vi "LV SciSDK ADD BOARD.vi"(5 "JsonFile":path, 7 "Board Model":string(combo), 8 "error in (no error)":errorcluster, 9 "handle":u64, 10 "DevicePath":string, 11 "Name":string) -> (0 "error out":errorcluster, 3 "handle":T1)   [LabVIEW 2021]
uses:
  SciSDK_Labview.lvlib
panel:
  out "Add device result":i32
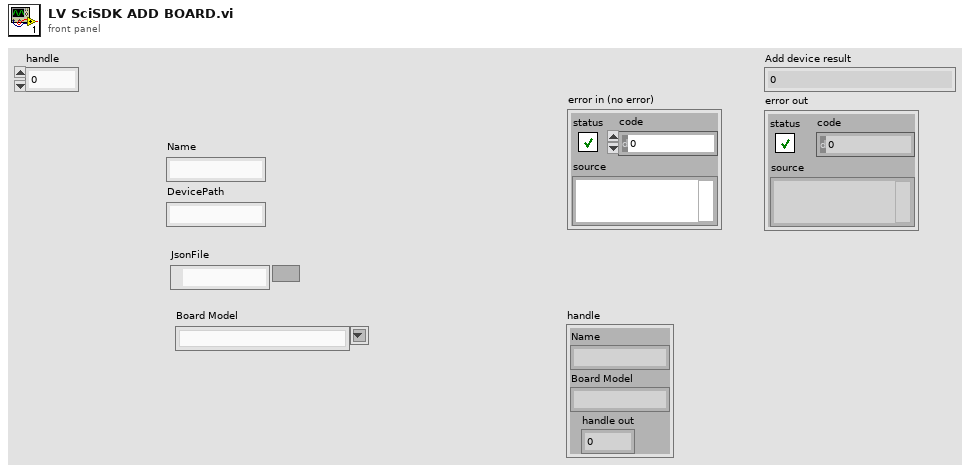
[diagram p1: front panel]
types:
  T1 = cluster{"Name":string, "Board Model":string, "handle out":u64}
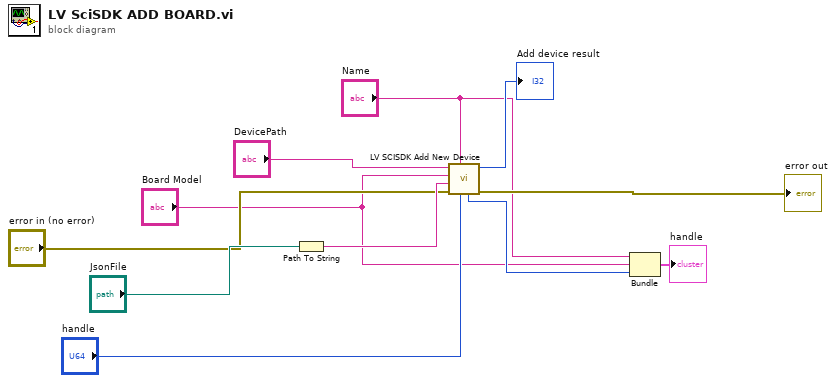
[diagram p0: block diagram]
diagram:
  n1 = Path To String(path="JsonFile") -> (string=w8:string)
  n2 = call "LV SCISDK Add New Device.vi"("handle"="handle", "Name"="Name", "error in (no error)"="error in (no error)", "JSONFwFilePath"=w8, "DeviceModel"="Board Model", "DevicePath"="DevicePath") -> ("error out"=→"error out":errorcluster, "function return"=→"Add device result":i32, "handle out"=w4:u64)  [unwired: 3 in]
  n3 = Bundle("Name"="Name", "Board Model"="Board Model", "handle out"=w4) -> (→"handle":T1)  [unwired: 1 in]
